vi "Set Char Size.vi"(5 "widh (same as height)":sgl, 7 "height":sgl=16.0, 8 "error in (no error)":errorcluster, 9 "v_res":u32=300, 10 "h_res":u32=300, 11 "face in":i64) -> (0 "error out":errorcluster, 3 "face out":i64)   [LabVIEW 2023, in "Freetype Drawer.lvlib"]
uses:
  Freetype Drawer.lvlib
  libfreetype.dll
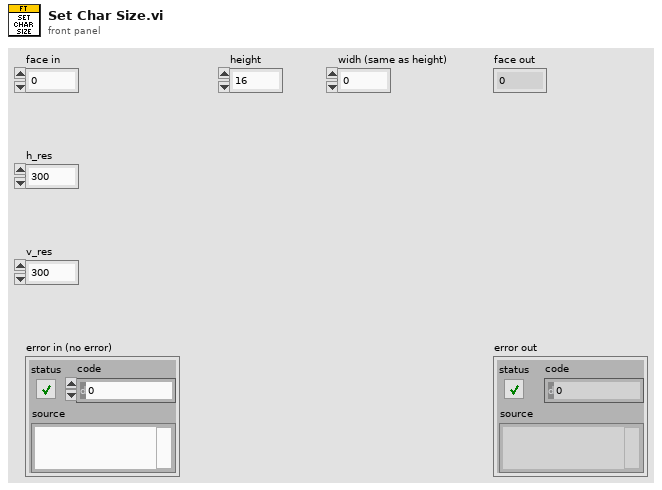
[diagram p1: front panel]
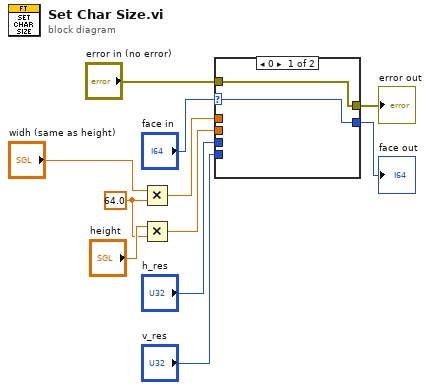
[diagram p0: block diagram]
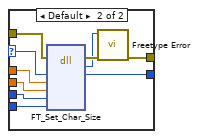
[diagram p2: hidden frame]
diagram:
  w8 = sgl 64.0 ("y")
  n1 = Multiply(x="widh (same as height)", y=w8) -> (x*y=w7:sgl)
  n2 = Multiply(x="height", y=w8) -> (x*y=w10:sgl)
  n3 = case shown="0" "face in" {
    selector: "face in" -> [w12 w21]
    tunnel: w10 -> [_ w23]
    tunnel: w7 -> [_ w22]
    tunnel: [w12 w20] -> w5
    tunnel: "error in (no error)" -> [w13 w19]
    tunnel: "h_res" -> [_ w18]
    tunnel: "v_res" -> [_ w17]
    tunnel: [w13 w14] -> w1
    frame 0 {
    }
    frame Default {
      n4 = dll-call lib="E:/Labview/LV 2023/Libs/LV Symbol/Freetype Drawer/libfreetype.dll" fn="FT_Set_Char_Size"(error in=w19, "face"=w21, "width"=w22, "height"=w23, "h_res"=w18, "v_res"=w17) -> (error out=w16:errorcluster, "error"=w15:i32, "face"=w20:i64)  [unwired: 6 in, 1 out]
      n5 = call "Freetype Error.vi"("error in (no error)"=w16, "Error"=w15) -> ("error out"=w14:errorcluster)  [unwired: 9 in]
    }
  }
  "face out" <- w5
  "error out" <- w1
